vi "SET_FIRE_PRESET.vi"(10 "argv":string[](array[string]), 11 "args":u8) -> ()   [LabVIEW 2011]
uses:
  gun/gun_tracking_mode.ctl
  <vilib>/Rock Robotics/WPI/DriverStation/WPI_DriverStationStatusErrorCache.ctl
  signals/Signal.ctl
  Auto_Conf.vi
panel:
  in  "StateMaps":cluster{"Name":string, "State":T1}[](array[cluster])=[{"Name"="auto_aim_camera", "State"=enum."auto_aim_camera"}, {"Name"="preset_center_field", "State"=enum."preset_center_field"}, {"Name"="preset_right_pocket", "State"=enum."preset_right_pocket"}, {"Name"="preset_left_pocket", "State"=enum."preset_left_pocket"}, {"Name"="align_center", "State"=enum."align_center"}, {"Name"="align_center_backward", "State"=enum."align_center_backwards"}, {"Name"="align_fold", "State"=enum."align_fold"}, {"Name"="auto_aim_key", "State"=enum."auto_aim_auton"}, {"Name"="auton_custom", "State"=enum."auton_custom"}]
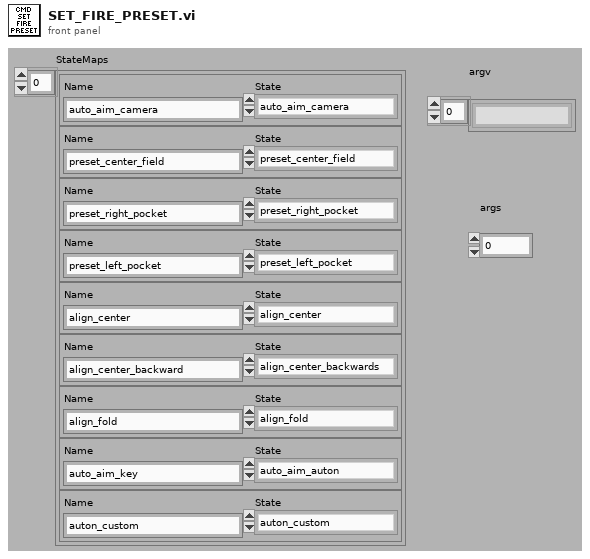
[diagram p1: front panel]
types:
  T1 = typedef "gun_tracking_mode.ctl" = enum16{"manual_aim", "auto_aim_camera", "preset_center_field", "preset_right_pocket", "preset_left_pocket", "align_center", "align_center_backwards", "auto_aim_key", "align_fold", "auton_custom", "preset_pass", "auto_aim_auton"}
  T2 = typedef "WPI_DriverStationStatusErrorCache.ctl" = enum16{"Get", "Set"}
  T3 = typedef "Signal.ctl" = enum16{"SIGFIRE", "SIGSTOPSCRIPT", "SIGSTARTGUN", "SIGSTOPGUN", "SIGDISABLED", "SIGENABLED", "SIGUDPTIMEOUT", "SIGNEWVISION_REMOTE", "SIGNEWVISION_LOCAL", "SIGSHOTFIRED", "SIGDOTRACK", "SIGDONTTRACK"}
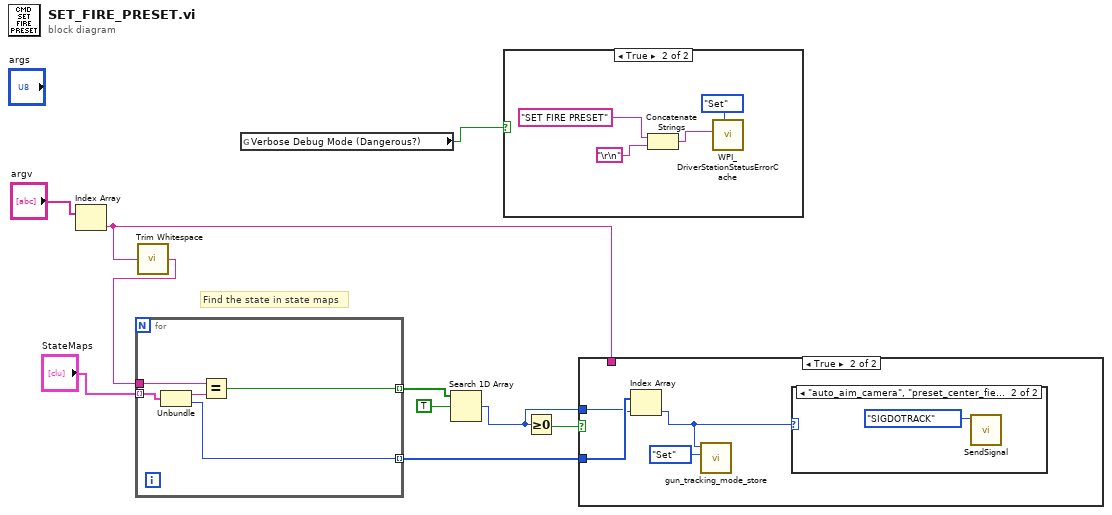
[diagram p0: block diagram]
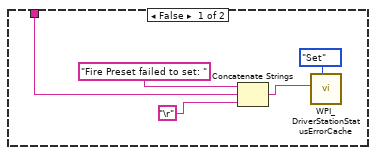
[diagram p3: hidden frame]
diagram:
  # "Find the state in state maps"
  n1 = Index Array(array="argv") -> (element=w2:string)  [unwired: 1 in]
  n2 = call <vilib>:"Trim Whitespace.vi"("string"=w2) -> ("trimmed string"=w1:string)  [unwired: 1 in]
  n3 = for {
    tunnel: w1 -> [w15]
    tunnel: "StateMaps" -> [w14] mode=indexing
    tunnel: [w12] -> w8 mode=indexing
    tunnel: [w11] -> w5 mode=indexing
    n4 = Unbundle(w14) -> ("Name"=w13:string, "State"=w11:T1)
    n5 = Equal?(x=w15, y=w13) -> (x = y?=w12:bool)
  }
  n6 = global read "Auto_Conf.vi" "Verbose Debug Mode (Dangerous?)"() -> (w3:bool)
  n7 = Search 1D Array(1D array=w8, element=TRUE) -> (index of element=w4:i32)  [unwired: 1 out]
  n8 = case shown="True" w3 {
    frame False {
    }
    frame True {
      n9 = Concatenate Strings("SET FIRE PRESET" ("string"), "\r\n") -> (w17:string)
      n10 = call <vilib>:"WPI_DriverStationStatusErrorCache.vi"("StatusErrorCacheOp"=WPI_DriverStationStatusErrorCache."Set", "Error String"=w17) -> ()  [unwired: 10 out]
    }
  }
  n11 = Greater Or Equal To 0?(x=w4) -> (x >= 0?=w6:bool)
  n12 = case shown="True" w6 {
    tunnel: w5 -> [_ w28]
    tunnel: w4 -> [_ w27]
    tunnel: w2 -> [w21 _]
    frame False {
      n13 = Concatenate Strings("Fire Preset failed to set: " ("string"), w21, "\r") -> (w22:string)
      n14 = call <vilib>:"WPI_DriverStationStatusErrorCache.vi"("StatusErrorCacheOp"=WPI_DriverStationStatusErrorCache."Set", "Error String"=w22) -> ()  [unwired: 10 out]
    }
    frame True {
      n15 = Index Array(array=w28, index=w27) -> (element=w25:T1)
      n16 = call "gun_tracking_mode_store.vi"("data_store_mode"=enum16{"Set", "Get"}."Set", "gun tracking mode"=w25) -> ()  [unwired: 9 in, 1 out]
      n17 = case shown="\"auto_aim_camera\", \"preset_center_field\", \"auto_aim_key\"" w25 {
        frame Default {
        }
        frame "auto_aim_camera", "preset_center_field", "auto_aim_key" {
          n18 = call "SendSignal.vi"("Signal"=Signal."SIGDOTRACK") -> ()  [unwired: 11 in]
        }
      }
    }
  }
